vi "Demo2.vi"() -> ()   [LabVIEW 2014]
uses:
  1/ExampleClass.lvclass
  2/ExampleClass2.lvclass
  2/ExampleClass2.lvclass/ExampleClass2.ctl
  1/ExampleClass.lvclass/ExampleClass.ctl
  Singleton/Singleton.lvclass
panel:
  in  "stop":bool
  out "Numeric 3":dbl
  out "created new? 4":bool
  out "created new? 3":bool
  out "Numeric 2":dbl
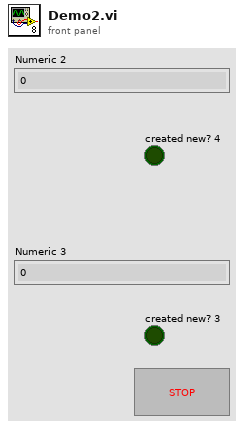
[diagram p1: front panel]
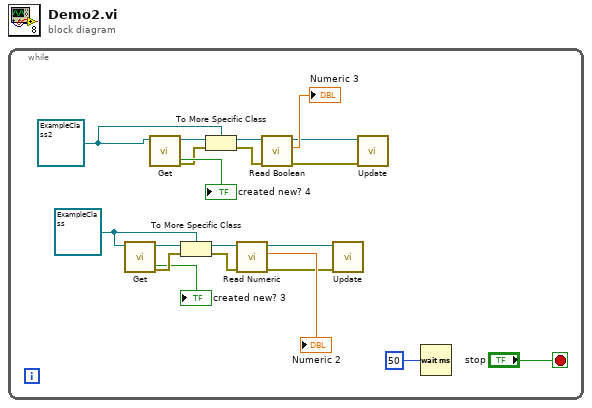
[diagram p0: block diagram]
diagram:
  n1 = while {
    stop <- "stop" stop-if-true
    w16 = refnum<class "ExampleClass2.lvclass"> refnum ("ExampleClass2")
    w6 = refnum<class "ExampleClass.lvclass"> refnum ("ExampleClass")
    n2 = call "Get.vi"("Template"=w6) -> ("error out"=w8:errorcluster, "object"=w2:refnum<class "Singleton.lvclass">, "created new?"=→"created new? 3":bool)  [unwired: 8 in]
    n3 = call "Get.vi"("Template"=w16) -> ("error out"=w11:errorcluster, "object"=w14:refnum<class "Singleton.lvclass">, "created new?"=→"created new? 4":bool)  [unwired: 8 in]
    n4 = To More Specific Class(target class=w6, reference=w2, error in=w8) -> (specific class reference=w5:refnum<class "ExampleClass.lvclass">, error out=w9:errorcluster)
    n5 = To More Specific Class(target class=w16, reference=w14, error in=w11) -> (specific class reference=w17:refnum<class "ExampleClass2.lvclass">, error out=w10:errorcluster)
    n6 = call "Read Numeric.vi"("error in (no error)"=w9, "ExampleClass in"=w5) -> ("error out"=w1:errorcluster, "Numeric"=→"Numeric 2":dbl, "ExampleClass out"=w3:refnum<class "ExampleClass.lvclass">)  [unwired: 7 in]
    n7 = call "Read Boolean.vi"("error in (no error)"=w10, "ExampleClass2 in"=w17) -> ("error out"=w15:errorcluster, "Numeric"=→"Numeric 3":dbl, "ExampleClass2 out"=w13:refnum<class "ExampleClass2.lvclass">)  [unwired: 7 in]
    n8 = call "Update.vi"("error in (no error)"=w1, "Object"=w3) -> ()  [unwired: 7 in, 3 out]
    n9 = call "Update.vi"("error in (no error)"=w15, "Object"=w13) -> ()  [unwired: 7 in, 3 out]
    n10 = Wait (ms)(milliseconds to wait=u32 50) -> ()  [unwired: 1 out]
  }
